vi "dB.vi"(3 "error in (no error)":errorcluster, 5 "Potencia":dbl) -> (0 "dBm":dbl, 1 "error out":errorcluster, 2 "dBW":dbl)   [LabVIEW 2019]
doc: "Calculo de dBW y dBm de la potencia de entrada en W"
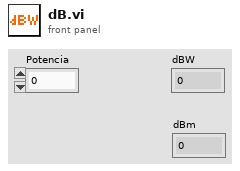
[diagram p1: front panel]
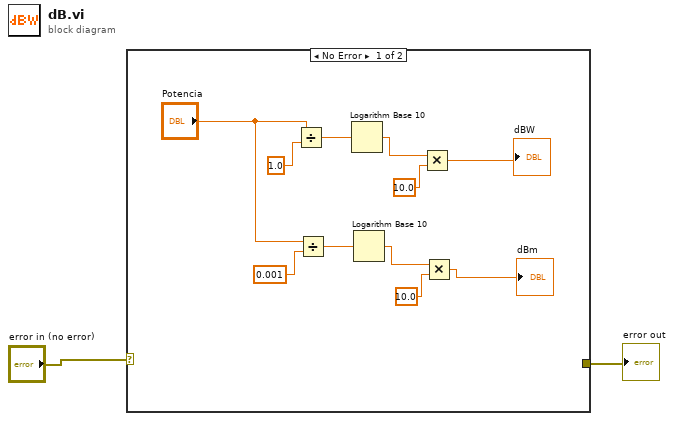
[diagram p0: block diagram]
diagram:
  n1 = case shown="No Error" "error in (no error)" {
    selector: "error in (no error)" -> [_ w14]
    tunnel: [_ w14] -> w1
    frame No Error {
      n2 = Divide(x="Potencia", y=1.0) -> (x/y=w12:dbl)
      n3 = Divide(x="Potencia", y=0.001) -> (x/y=w6:dbl)
      n4 = Logarithm Base 10(1:w12) -> (0:w11:dbl)
      n5 = Logarithm Base 10(1:w6) -> (0:w7:dbl)
      n6 = Multiply(x=w11, y=10.0) -> (x*y=→"dBW":dbl)
      n7 = Multiply(x=w7, y=10.0) -> (x*y=→"dBm":dbl)
    }
    frame Error {
    }
  }
  "error out" <- w1
